vi "Data.vi"(8 "error in (no error)":errorcluster, 11 "PB Msg Template in":refnum<class "Msg.lvclass">) -> (0 "error out":errorcluster, 2 "Data":T1, 3 "PB Msg Template out":refnum<class "Msg.lvclass">)   [LabVIEW 2020, in "TcpAckNack.lvlib" / "Msg.lvclass"]
uses:
  Msg.lvclass
  Data.ctl
  TcpAckNack.lvlib
  AckNackResult/Enumeration.ctl
  AckNackResult/AckNackResult.lvlib
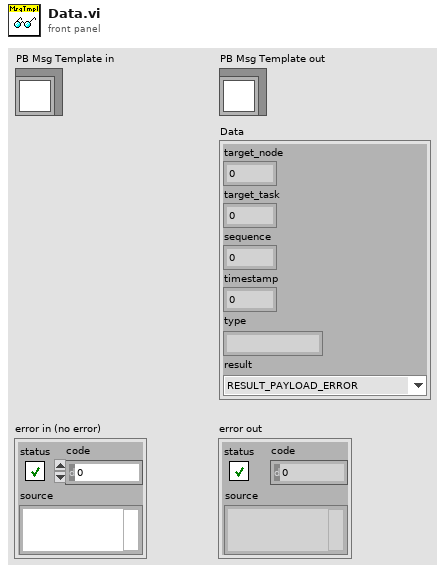
[diagram p1: front panel]
types:
  T1 = typedef "TcpAckNack.lvlib/Data.ctl" = cluster{"target_node":u32, "target_task":u32, "sequence":u32, "timestamp":u64, "type":string, "result":T2}
  T2 = typedef "AckNackResult.lvlib/Enumeration.ctl" = enum16{"RESULT_PAYLOAD_ERROR", "RESULT_UNEXPECTED_TYPE", "RESULT_EXPIRED", "RESULT_OUTOFSEQUENCE", "RESULT_DISALLOWED", "RESULT_INVALIDTASK", "RESULT_INVALIDTARGET", "RESULT_UNKNOWN", "RESULT_ACK"}
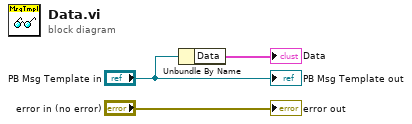
[diagram p0: block diagram]
diagram:
  n1 = Unbundle By Name("PB Msg Template in") -> ("Data"=→"Data":T1)
  "error out" <- "error in (no error)"
  "PB Msg Template out" <- "PB Msg Template in"
